vi "4-3.vi"(1 "数值":i32) -> (0 "sqrt(x)":dbl)   [LabVIEW 2017]
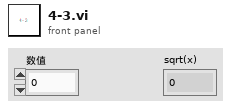
[diagram p1: front panel]
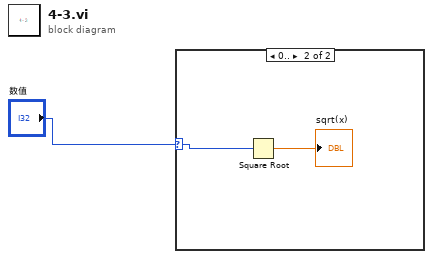
[diagram p0: block diagram]
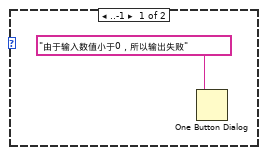
[diagram p2: hidden frame]
diagram:
  n1 = case shown="0.." "数值" {
    selector: "数值" -> [_ w4]
    frame ..-1 {
      n2 = One Button Dialog(message="由于输入数值小于0，所以输出失败") -> ()  [unwired: 1 in, 1 out]
    }
    frame 0.. {
      n3 = Square Root(x=w4) -> (sqrt(x)=→"sqrt(x)":dbl)
    }
  }
